vi "ScanDelay_FTIR_InterferogramDAQmxTask.vi"(6 "First clear existing DAQmx tasks":bool=TRUE, 8 "Channels to read":tag="Dev1/ai2,Dev1/ai3", 9 "Sampling rate":dbl=250000.0, 10 "Time per acquisiton (s)":dbl=0.18, 11 "Trigger Terminal":tag="/Dev1/PFI0") -> (0 "error out":errorcluster={"status"=TRUE, "code"=-50103, "source"="DAQmx Control Task.vi:3900001<append>\n<B>Task Name: </B>_unnamedTask<C5532>"}, 3 "Refnum out":refnum<k21>)   [LabVIEW 2022 SP3]
uses:
  <vilib>/DAQmx/create/channels.llb/DAQmx Create Channel (AI-Voltage-Basic).vi
  <vilib>/DAQmx/configure/timing.llb/DAQmx Timing (Sample Clock).vi
  <vilib>/DAQmx/configure/trigger.llb/DAQmx Start Trigger (Digital Edge).vi
  <resource>/objmgr/daqmx.rc
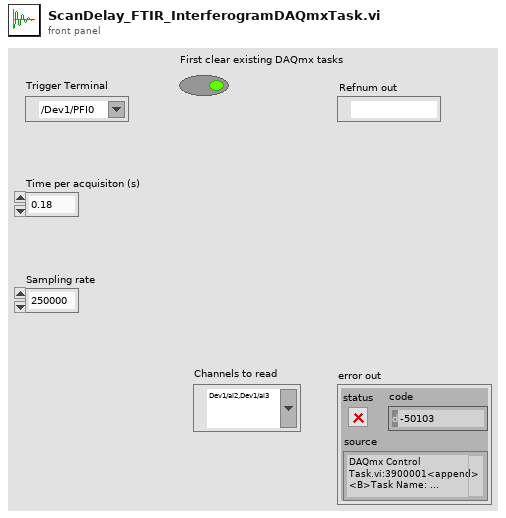
[diagram p1: front panel]
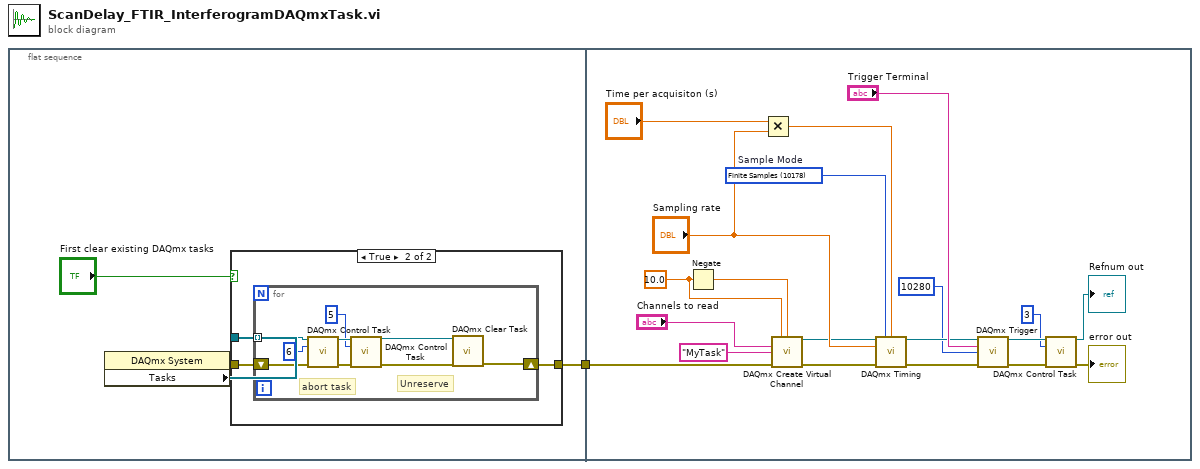
[diagram p0: block diagram]
diagram:
  n1 = flat-sequence {
    tunnel: [w2] -> w1
    tunnel: w1 -> [w19]
    frame #0 {
      n2 = property class="DAQmx System"() -> (error out=w3:errorcluster, "Tasks"=w4:refnum<k21>[])  [unwired: 2 in, 1 out]
      n3 = case shown="True" "First clear existing DAQmx tasks" {
        tunnel: w4 -> [_ w9]
        tunnel: w3 -> [w6 w8]
        tunnel: [w6 w7] -> w2
        frame False {
        }
        frame True {
          n4 = for {
            tunnel: w9 -> [w18] mode=indexing
            shift-right: [w11] -> w7
            shift-left: w8 -> [w16]
            # "abort task"
            # "Unreserve"
            n5 = call <vilib>:"DAQmx Control Task.vi"("task/channels in"=w18, "action"=6, "error in"=w16) -> ("task out"=w17:refnum<k21>, "error out"=w15:errorcluster)  [unwired: 11 in]
            n6 = call <vilib>:"DAQmx Control Task.vi"("task/channels in"=w17, "action"=5, "error in"=w15) -> ("task out"=w10:refnum<k21>, "error out"=w12:errorcluster)  [unwired: 11 in]
            n7 = call <vilib>:"DAQmx Clear Task.vi"("task in"=w10, "error in"=w12) -> ("error out"=w11:errorcluster)  [unwired: 13 in]
          }
        }
      }
    }
    frame #1 {
      w34 = 10178 items=["Finite Samples"=10178, "Continuous Samples"=10123, "Hardware Timed Single Point"=12522]  # Sample Mode
      w31 = 10.0
      n8 = Negate(x=w31) -> (-x=w32:dbl)
      n9 = Multiply(x="Time per acquisiton (s)", y="Sampling rate") -> (x*y=w25:dbl)
      n10 = call-poly <vilib>:"DAQmx Create Virtual Channel.vi"("maximum value"=w31, "minimum value"=w32, "physical channels"="Channels to read", "name to assign"="MyTask", "error in"=w19) -> ("task out"=w33:refnum<k21>, "error out"=w35:errorcluster)  [unwired: 9 in]
      n11 = call-poly <vilib>:"DAQmx Timing.vi"("task/channels in"=w33, "sample mode"=w34, "samples per channel"=w25, "rate"="Sampling rate", "error in"=w35) -> ("task out"=w29:refnum<k21>, "error out"=w38:errorcluster)  [unwired: 9 in]
      n12 = call-poly <vilib>:"DAQmx Trigger.vi"("task/channels in"=w29, "source"="Trigger Terminal", "edge"=10280, "error in"=w38) -> ("task out"=w24:refnum<k21>, "error out"=w21:errorcluster)  [unwired: 10 in]
      n13 = call <vilib>:"DAQmx Control Task.vi"("task/channels in"=w24, "action"=3, "error in"=w21) -> ("task out"=→"Refnum out":refnum<k21>, "error out"=→"error out":errorcluster)  [unwired: 11 in]
    }
  }
